vi "Check Value.vi"(6 "Coerce Value? (F)":bool, 7 "Column Configuration":refnum<class "Column Configuration.lvclass">, 8 "error in (no error)":errorcluster, 9 "Value Type":refnum<class "Value Type.lvclass">, 10 "Value In":variant, 11 "Check in":refnum<class "Constraint.lvclass">) -> (0 "error out":errorcluster, 2 "Value Out":variant, 3 "Check out":refnum<class "Constraint.lvclass">)   [LabVIEW 2020, in "Composed Columns.lvlib" / "Constraint.lvclass"]
uses:
  Constraint.lvclass
  Value Type/Value Type.lvclass
  Basic Columns/Column Configuration/Basic Column Configuration Class/Column Configuration.lvclass
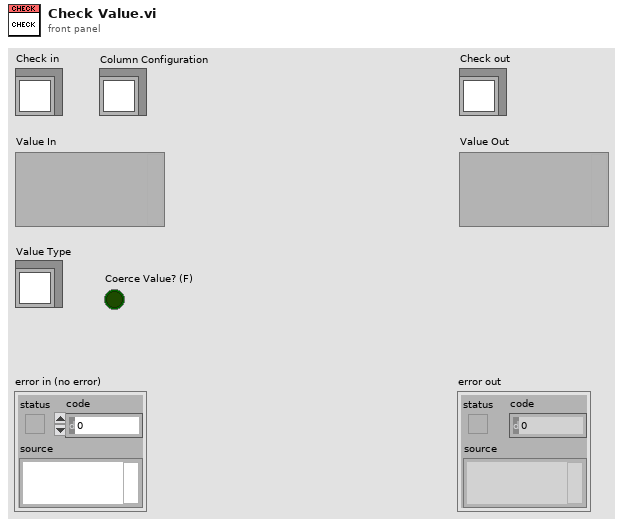
[diagram p1: front panel]
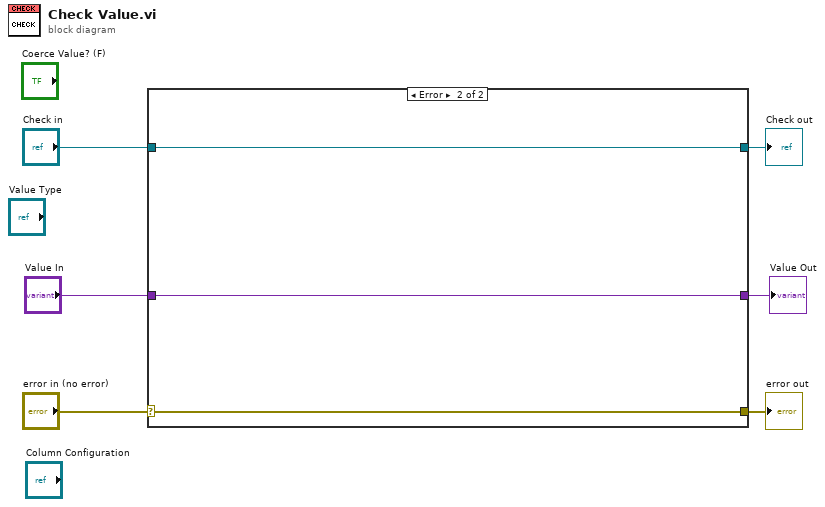
[diagram p0: block diagram]
diagram:
  n1 = case shown="Error" "error in (no error)" {
    selector: "error in (no error)" -> [w8 w12]
    tunnel: [w8 w12] -> w5
    tunnel: [w9 w11] -> w3
    tunnel: "Check in" -> [w9 w11]
    tunnel: "Value In" -> [w7 w10]
    tunnel: [w7 w10] -> w1
    frame No Error {
      # "Wire the error cluster across even in the \"No Error\"\ncase so that warnings get propagated."
    }
    frame Error {
    }
  }
  "error out" <- w5
  "Check out" <- w3
  "Value Out" <- w1
